vi "Compute Layout.vi"(0 "State":T1={"Nspeakers"=13, "actions"=[], "Wspeaker"=13, "hover"={"type"=enum."None", "index"=0}, "locked"=FALSE, "states"=[], "sel speak"=13, "selected"=refnum, "Events"={"Selection change"=refnum}}, 5 "picture ref":refnum<vi>, 7 "Size":i32) -> (4 "Layout":T6, 6 "Wpict":u32, 8 "Hpict":u32, 10 "Hcontrol":u32)   [LabVIEW 2020, in "SAC Config.xctl"]
uses:
  SAC Config.xctl
  Layout.ctl
  Item.ctl
  State.vi
  Hover Data.ctl
  Hover Item.ctl
  Speaker State.ctl
  Events.ctl
  Selection changed.ctl
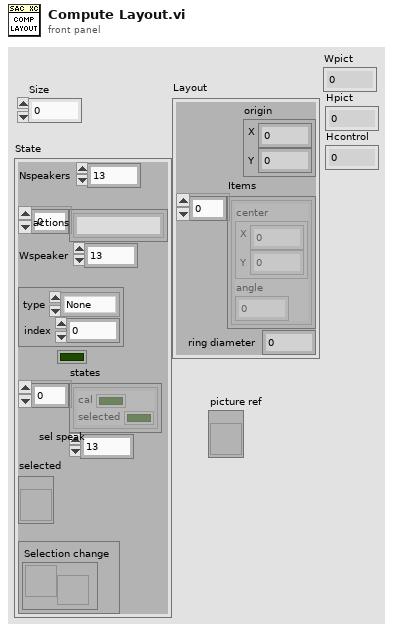
[diagram p1: front panel]
types:
  T1 = typedef "SAC Config.xctl/State.vi" = cluster{"Nspeakers":i32, "actions":string[], "Wspeaker":i32, "hover":T2, "locked":bool, "states":T4[], "sel speak":i32, "selected":refnum<vi>, "Events":T5}
  T2 = typedef "SAC Config.xctl/Hover Data.ctl" = cluster{"type":T3, "index":i32}
  T3 = typedef "SAC Config.xctl/Hover Item.ctl" = enum16{"None", "Speaker"}
  T4 = typedef "SAC Config.xctl/Speaker State.ctl" = cluster{"cal":bool, "selected":bool}
  T5 = typedef "SAC Config.xctl/Events.ctl" = cluster{"Selection change":refnum<user-event>}
  T6 = typedef "SAC Config.xctl/Layout.ctl" = cluster{"origin":cluster{"X":i32, "Y":i32}, "Items":T7[], "ring diameter":i32}
  T7 = typedef "SAC Config.xctl/Item.ctl" = cluster{"center":cluster{"X":i32, "Y":i32}, "angle":dbl}
  T8 = typedef "LVBoundsTypeDef.ctl" = cluster{"Width":u32, "Height":u32}
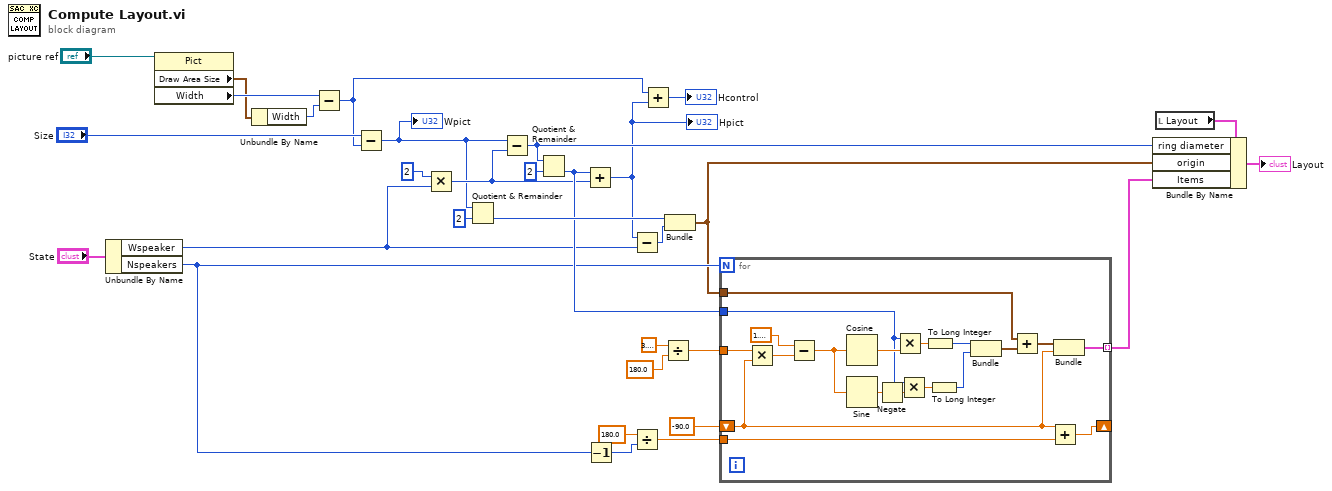
[diagram p0: block diagram]
diagram:
  n1 = Unbundle By Name("State") -> ("Wspeaker"=w8:i32, "Nspeakers"=w2:i32)
  n2 = property class="Pict"(reference="picture ref") -> ("Draw Area Size"=w11:T8, "Width"=w12:u32)  [unwired: 1 in, 2 out]
  n3 = Unbundle By Name(w11) -> ("Width"=w13:u32)
  n4 = Subtract(x=w12, y=w13) -> (x-y=w4:u32)
  n5 = Subtract(x="Size", y=w4) -> (x-y=w6:u32)
  "Wpict" <- w6
  n6 = Multiply(x=2 ("y"), y=w8) -> (x*y=w14:i32)
  n7 = Quotient & Remainder(x=w6, y=2) -> (floor(x/y)=w20:u32)  [unwired: 1 out]
  n8 = Subtract(x=w6, y=w14) -> (x-y=w7:u32)
  n9 = Quotient & Remainder(x=w7, y=2) -> (floor(x/y)=w18:u32)  [unwired: 1 out]
  n10 = Add(x=w18, y=w14) -> (x+y=w5:u32)
  "Hpict" <- w5
  n11 = Decrement(x=w2) -> (x-1=w16:i32)
  n12 = Subtract(x=w5, y=w8) -> (x-y=w27:u32)
  n13 = Divide(x=180.0, y=w16) -> (x/y=w25:dbl)
  n14 = Add(x=w4, y=w5) -> (x+y=→"Hcontrol":u32)
  n15 = Divide(x=3.141592653589793, y=180.0) -> (x/y=w22:dbl)
  n16 = Bundle(w20, w27) -> (w1:cluster{u32, u32})  [unwired: 1 in]
  n17 = for {
    N: w2 -> [_]
    tunnel: w1 -> [w36]
    shift-right: [w50] -> _
    shift-left: -90.0 -> [w39]
    tunnel: w25 -> [w49]
    tunnel: w22 -> [w48]
    tunnel: w18 -> [w44]
    tunnel: [w38] -> w21 mode=indexing
    n18 = Multiply(x=w48, y=w39) -> (x*y=w35:dbl)
    n19 = Subtract(x=1.5707963267948966, y=w35) -> (x-y=w34:dbl)
    n20 = Cosine(x=w34) -> (cos(x)=w47:dbl)
    n21 = Sine(x=w34) -> (sin(x)=w43:dbl)
    n22 = Negate(x=w43) -> (-x=w32:dbl)
    n23 = Multiply(x=w44, y=w47) -> (x*y=w46:dbl)
    n24 = Multiply(x=w44, y=w32) -> (x*y=w45:dbl)
    n25 = To Long Integer(number=w46) -> (32bit integer=w42:i32)
    n26 = To Long Integer(number=w45) -> (32bit integer=w41:i32)
    n27 = Bundle(w42, w41) -> (w40:cluster{i32, i32})  [unwired: 1 in]
    n28 = Add(x=w36, y=w40) -> (x+y=w37:cluster{u32, u32})
    n29 = Add(x=w39, y=w49) -> (x+y=w50:dbl)
    n30 = Bundle(w37, w39) -> (w38:cluster{cluster{u32, u32}, dbl})  [unwired: 1 in]
  }
  n31 = local read "Layout"() -> (w30:T6)
  n32 = Bundle By Name(cluster=w30, "ring diameter"=w7, "origin"=w1, "Items"=w21) -> (→"Layout":T6)
